vi "11.2.4.-Momento Invariante de Hu Normalizado - Npq.vi"(0 "u00":dbl, 1 "u11":dbl, 2 "u12":dbl, 3 "u02":dbl, 4 "u20":dbl, 5 "u21":dbl, 6 "u03":dbl, 7 "u30":dbl) -> (20 "n11":dbl, 21 "n12":dbl, 22 "n02":dbl, 23 "n20":dbl, 24 "n21":dbl, 25 "n03":dbl, 26 "n30":dbl)   [LabVIEW 2020]
panel:
  # "Visión Artificial - Momentos Invariantes de Hu\nDiego Cervantes Rodríguez\ndicer0.com"
  # "Momento normalizado = Npq = Upq/u00^d, donde:\nd = ((p+q)/2)+1, si p+q > 1\nd = 1, si p+q <= 1"
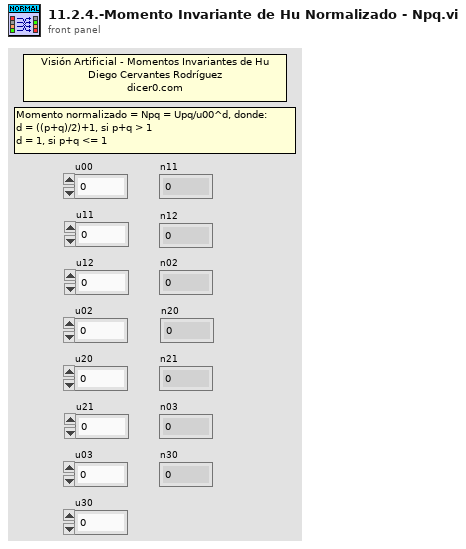
[diagram p1: front panel]
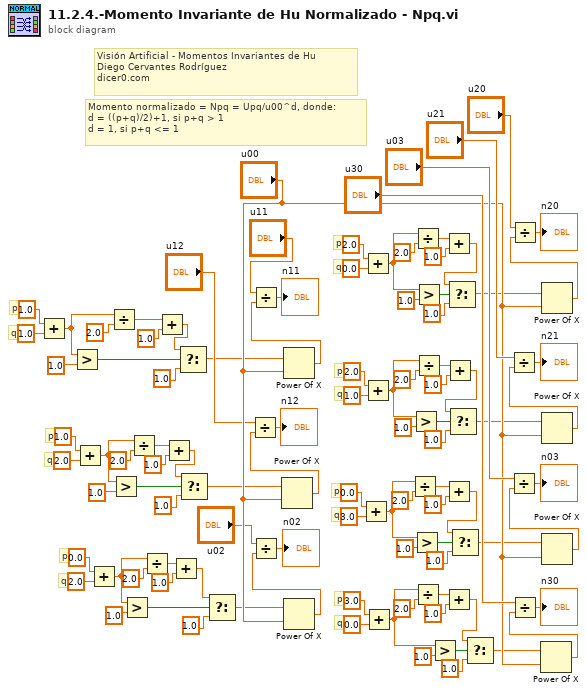
[diagram p0: block diagram]
diagram:
  # "Momento normalizado = Npq = Upq/u00^d, donde:\nd = ((p+q)/2)+1, si p+q > 1\nd = 1, si p+q <= 1"
  # "Visión Artificial - Momentos Invariantes de Hu\nDiego Cervantes Rodríguez\ndicer0.com"
  # "q"
  # "p"
  # "q"
  # "p"
  # "q"
  # "p"
  # "q"
  # "p"
  # "q"
  # "p"
  # "q"
  # "p"
  # "q"
  # "p"
  n1 = Add(x=1.0, y=1.0) -> (x+y=w19:dbl)
  n2 = Greater?(x=w19, y=1.0) -> (0:w21:bool)
  n3 = Add(x=1.0, y=2.0) -> (x+y=w9:dbl)
  n4 = Add(x=0.0, y=2.0) -> (x+y=w31:dbl)
  n5 = Divide(x=w19, y=2.0) -> (x/y=w17:dbl)
  n6 = Greater?(x=w9, y=1.0) -> (0:w11:bool)
  n7 = Greater?(x=w31, y=1.0) -> (0:w33:bool)
  n8 = Divide(x=w9, y=2.0) -> (x/y=w7:dbl)
  n9 = Divide(x=w31, y=2.0) -> (x/y=w29:dbl)
  n10 = Add(x=w17, y=1.0) -> (x+y=w16:dbl)
  n11 = Add(x=w7, y=1.0) -> (x+y=w6:dbl)
  n12 = Add(x=w29, y=1.0) -> (x+y=w28:dbl)
  n13 = Select(t=w16, s=w21, f=1.0) -> (s? t:f=w4:dbl)
  n14 = Select(t=w6, s=w11, f=1.0) -> (s? t:f=w2:dbl)
  n15 = Select(t=w28, s=w33, f=1.0) -> (s? t:f=w26:dbl)
  n16 = Power Of X(1:"u00", 2:w2) -> (0:w1:dbl)
  n17 = Divide(x="u12", y=w1) -> (x/y=→"n12":dbl)
  n18 = Power Of X(1:"u00", 2:w4) -> (0:w3:dbl)
  n19 = Divide(x="u11", y=w3) -> (x/y=→"n11":dbl)
  n20 = Power Of X(1:"u00", 2:w26) -> (0:w25:dbl)
  n21 = Divide(x="u02", y=w25) -> (x/y=→"n02":dbl)
  n22 = Add(x=0.0, y=3.0) -> (x+y=w73:dbl)
  n23 = Add(x=2.0, y=0.0) -> (x+y=w61:dbl)
  n24 = Add(x=2.0, y=1.0) -> (x+y=w51:dbl)
  n25 = Add(x=3.0, y=0.0) -> (x+y=w88:dbl)
  n26 = Divide(x=w73, y=2.0) -> (x/y=w71:dbl)
  n27 = Greater?(x=w51, y=1.0) -> (0:w53:bool)
  n28 = Greater?(x=w73, y=1.0) -> (0:w75:bool)
  n29 = Divide(x=w61, y=2.0) -> (x/y=w59:dbl)
  n30 = Divide(x=w88, y=2.0) -> (x/y=w86:dbl)
  n31 = Greater?(x=w61, y=1.0) -> (0:w63:bool)
  n32 = Divide(x=w51, y=2.0) -> (x/y=w49:dbl)
  n33 = Greater?(x=w88, y=1.0) -> (0:w90:bool)
  n34 = Add(x=w59, y=1.0) -> (x+y=w58:dbl)
  n35 = Add(x=w71, y=1.0) -> (x+y=w70:dbl)
  n36 = Add(x=w86, y=1.0) -> (x+y=w85:dbl)
  n37 = Add(x=w49, y=1.0) -> (x+y=w48:dbl)
  n38 = Select(t=w58, s=w63, f=1.0) -> (s? t:f=w46:dbl)
  n39 = Select(t=w48, s=w53, f=1.0) -> (s? t:f=w44:dbl)
  n40 = Select(t=w70, s=w75, f=1.0) -> (s? t:f=w68:dbl)
  n41 = Select(t=w85, s=w90, f=1.0) -> (s? t:f=w83:dbl)
  n42 = Power Of X(1:"u00", 2:w83) -> (0:w82:dbl)
  n43 = Divide(x="u30", y=w82) -> (x/y=→"n30":dbl)
  n44 = Power Of X(1:"u00", 2:w46) -> (0:w45:dbl)
  n45 = Divide(x="u20", y=w45) -> (x/y=→"n20":dbl)
  n46 = Power Of X(1:"u00", 2:w44) -> (0:w43:dbl)
  n47 = Divide(x="u21", y=w43) -> (x/y=→"n21":dbl)
  n48 = Power Of X(1:"u00", 2:w68) -> (0:w67:dbl)
  n49 = Divide(x="u03", y=w67) -> (x/y=→"n03":dbl)
